vi "sample1(BasicRW PRO).vi"() -> ()   [LabVIEW 2020]
panel:
  in  "OffsetTime":u32=500
  out "err":errorcluster caption="エラー出力" {"code" format="%04x"}
  in  "ID":u8=1 max=253
  in  "Baudrate":u32=57600
  in  "COM":refnum<visa-resource-name> caption="COMポート"
  in  "STOP":bool
  in  "POSITION":i32(knob) min=-131594 max=131594 scale=100000.0..-100000.0
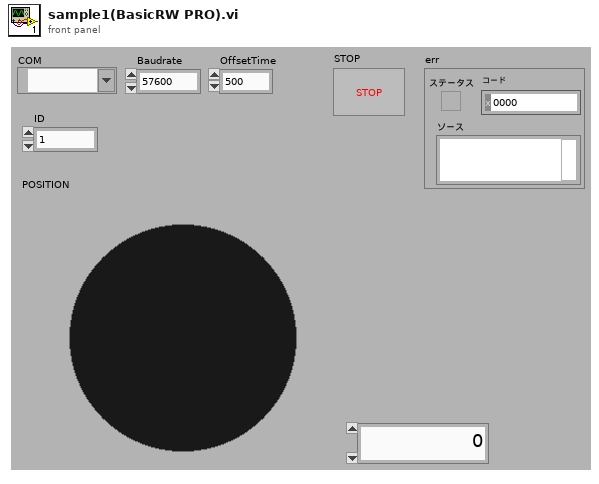
[diagram p1: front panel]
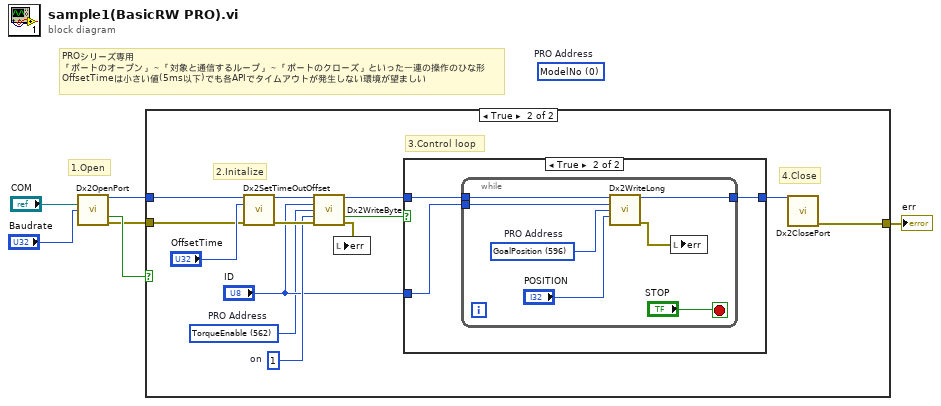
[diagram p0: block diagram]
diagram:
  (unwired) u16 0 items=["ModelNo"=0, "ModelInfo"=2, "VersionOfFirmware"=6, "ID"=7, "Baudrate"=8, "ReturnDelayTime"=9, "OperationMode"=11, "HormingOffset"=13, "MovingThreshold"=17, "TemperatureLimit"=21, "MaxVoltageLimit"=22, "MinVoltageLimit"=24, "AccelerationLimit"=26, "TorqueLimit"=30, "VoltageLimit"=32, "MaxPositionLimit"=36, "MinPositionLimit"=40, "ExternalPortMode1"=44, "ExternalPortMode2"=45, "ExternalPortMode3"=46, "ExternalPortMode4"=47, "Shutdown"=48, "TorqueEnable"=562, "LED_Red"=563, "LED_Green"=564, "LED_Blue"=565, "VelocityIGain"=586, "VelocityPGain"=588, "PositionPGain"=594, "GoalPosition"=596, "GoalVelocity"=600, "GoalTorque"=604, "GoalAcceleration"=606, "Moving"=610, "PresentPosition"=611, "PresentVelocity"=615, "PresentCurrent"=621, "PresentInputVoltage"=623, "PresentTemperature"=625, "ExternalPortData1"=626, "ExternalPortData2"=628, "ExternalPortData3"=630, "ExternalPortData4"=632, "RegistedInstruction"=890, "StatusReturnLevel"=891, "HardwareError"=892]  # PRO Address
  # "1.Open"
  # "PROシリーズ専用\n「ポートのオープン」～「対象と通信するループ」～「ポートのクローズ」といった一連の操作のひな形\nOffsetTimeは小さい値(5ms以下)でも各APIでタイムアウトが発生しない環境が望ましい"
  n1 = call "Dx2OpenPort.vi"("port"="COM", "baudrate"="Baudrate") -> ("dvid"=w3:u32, "成功"=w4:bool, "エラー出力"=w2:errorcluster)  [unwired: 11 in]
  n2 = case shown="TRUE" w4 {
    tunnel: w3 -> [_ w20]
    tunnel: w2 -> [w7 w18]
    tunnel: [w7 w8] -> w1
    frame False {
      # "Fail to open"
    }
    frame True {
      w10 = u16 562 items=["ModelNo"=0, "ModelInfo"=2, "VersionOfFirmware"=6, "ID"=7, "Baudrate"=8, "ReturnDelayTime"=9, "OperationMode"=11, "HormingOffset"=13, "MovingThreshold"=17, "TemperatureLimit"=21, "MaxVoltageLimit"=22, "MinVoltageLimit"=24, "AccelerationLimit"=26, "TorqueLimit"=30, "VoltageLimit"=32, "MaxPositionLimit"=36, "MinPositionLimit"=40, "ExternalPortMode1"=44, "ExternalPortMode2"=45, "ExternalPortMode3"=46, "ExternalPortMode4"=47, "Shutdown"=48, "TorqueEnable"=562, "LED_Red"=563, "LED_Green"=564, "LED_Blue"=565, "VelocityIGain"=586, "VelocityPGain"=588, "PositionPGain"=594, "GoalPosition"=596, "GoalVelocity"=600, "GoalTorque"=604, "GoalAcceleration"=606, "Moving"=610, "PresentPosition"=611, "PresentVelocity"=615, "PresentCurrent"=621, "PresentInputVoltage"=623, "PresentTemperature"=625, "ExternalPortData1"=626, "ExternalPortData2"=628, "ExternalPortData3"=630, "ExternalPortData4"=632, "RegistedInstruction"=890, "StatusReturnLevel"=891, "HardwareError"=892]  # PRO Address
      w13 = u8 1  # on
      # "4.Close"
      # "3.Control loop"
      # "2.Initalize"
      n3 = call "Dx2SetTimeOutOffset.vi"("dvid in"=w20, "OffsetTime"="OffsetTime", "エラー入力"=w18) -> ("dvid out"=w17:u32, "エラー出力"=w15:errorcluster)  [unwired: 11 in]
      n4 = call "Dx2WriteByte.vi"("dvid in"=w17, "id"="ID", "address"=w10, "data in"=w13, "エラー入力"=w15) -> ("dvid out"=w14:u32, "成功"=w16:bool, "エラー出力"=w9:errorcluster)  [unwired: 8 in]
      n5 = local write "err"(w9) -> ()
      n6 = case shown="TRUE" w16 {
        tunnel: w14 -> [w21 w24]
        tunnel: "ID" -> [_ w23]
        tunnel: [w21 w22] -> w11
        frame False {
          # "Fail to initalize"
        }
        frame True {
          n7 = while {
            tunnel: w24 -> [w31]
            tunnel: w23 -> [w30]
            tunnel: [w28] -> w22
            stop <- "STOP" stop-if-true
            w26 = u16 596 items=["ModelNo"=0, "ModelInfo"=2, "VersionOfFirmware"=6, "ID"=7, "Baudrate"=8, "ReturnDelayTime"=9, "OperationMode"=11, "HormingOffset"=13, "MovingThreshold"=17, "TemperatureLimit"=21, "MaxVoltageLimit"=22, "MinVoltageLimit"=24, "AccelerationLimit"=26, "TorqueLimit"=30, "VoltageLimit"=32, "MaxPositionLimit"=36, "MinPositionLimit"=40, "ExternalPortMode1"=44, "ExternalPortMode2"=45, "ExternalPortMode3"=46, "ExternalPortMode4"=47, "Shutdown"=48, "TorqueEnable"=562, "LED_Red"=563, "LED_Green"=564, "LED_Blue"=565, "VelocityIGain"=586, "VelocityPGain"=588, "PositionPGain"=594, "GoalPosition"=596, "GoalVelocity"=600, "GoalTorque"=604, "GoalAcceleration"=606, "Moving"=610, "PresentPosition"=611, "PresentVelocity"=615, "PresentCurrent"=621, "PresentInputVoltage"=623, "PresentTemperature"=625, "ExternalPortData1"=626, "ExternalPortData2"=628, "ExternalPortData3"=630, "ExternalPortData4"=632, "RegistedInstruction"=890, "StatusReturnLevel"=891, "HardwareError"=892]  # PRO Address
            n8 = call "Dx2WriteLong.vi"("dvid in"=w31, "id"=w30, "address"=w26, "data in"="POSITION") -> ("dvid out"=w28:u32, "エラー出力"=w25:errorcluster)  [unwired: 9 in, 1 out]
            n9 = local write "err"(w25) -> ()
          }
        }
      }
      n10 = call "Dx2ClosePort.vi"("dvid"=w11) -> ("エラー出力"=w8:errorcluster)  [unwired: 13 in, 1 out]
    }
  }
  "err" <- w1
